vi "LC_frequenc.vi"() -> ()   [LabVIEW 2020]
panel:
  in  "stop":bool
  out "F":dbl
  in  "C":dbl(slide) scale=0.0..10.0
  in  "L":dbl(slide) scale=0.0..10.0
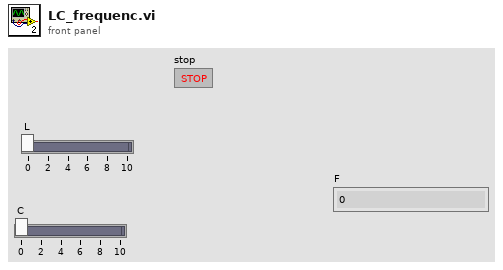
[diagram p1: front panel]
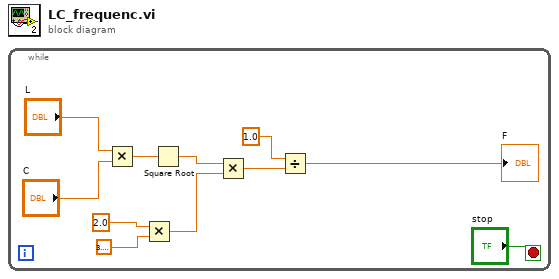
[diagram p0: block diagram]
diagram:
  n1 = while {
    stop <- "stop" stop-if-true
    n2 = Multiply(x="L", y="C") -> (x*y=w8:dbl)
    n3 = Multiply(x=2.0, y=3.141592653589793) -> (x*y=w4:dbl)
    n4 = Square Root(x=w8) -> (sqrt(x)=w7:dbl)
    n5 = Multiply(x=w7, y=w4) -> (x*y=w2:dbl)
    n6 = Divide(x=1.0, y=w2) -> (x/y=→"F":dbl)
  }
